vi "IMURead.vi"(10 "baud rate (57600)":u32=57600) -> (3 "Read":string)   [LabVIEW 2017]
uses:
  <vilib>/Instr/_visa.llb/VISA Configure Serial Port (Instr).vi
  <vilib>/Utility/error.llb/Error Cluster From Error Code.vi
  <vilib>/rvi/errors/niLvFpgaAdjustHostInterfaceError.vi
  <vilib>/FPGAPlugInAG/Dynamic/niLvFpga_Close_Dynamic.vi
  <vilib>/rvi/interface/nirviReadWriteControl/nirviReadWriteControl.xnode
  <vilib>/rvi/interface/nirviCloseFPGA/nirviCloseFPGA.xnode
  NiFpgaLv.dll
  <vilib>/rvi/interface/Simulation/niFpgaSimulationCallBeginRW.vi
panel:
  out "Other GSV":sgl
  out "Max Z Accel":sgl
  out "Max Y Accel":sgl
  out "Velocity GSV":dbl
  out "Y Velocity RAW":sgl
  out "Y Accel in m/s^2":sgl
  out "Z dTheta":sgl
  out "Y dTheta":sgl
  out "X dTheta":sgl
  out "Z Accel":sgl
  out "Y Accel":sgl
  out "X Accel":sgl
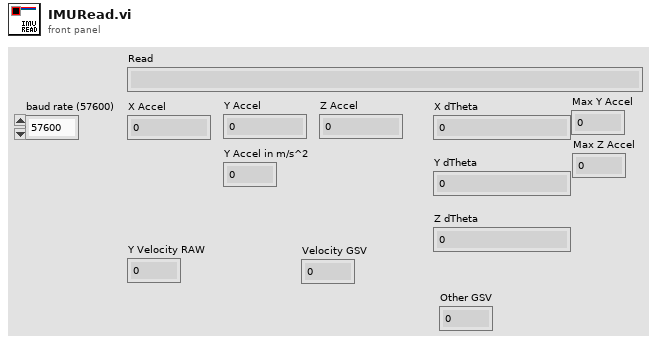
[diagram p1: front panel]
types:
  T1 = cluster{"X dtheta":sgl, "Y dtheta":sgl, "Z dtheta":sgl, "X accel":sgl, "Y accel":sgl, "Z accel":sgl, "Velocity":sgl, "IMU Fault":bool, "Time Since Last Tape":sgl, "Position":sgl}
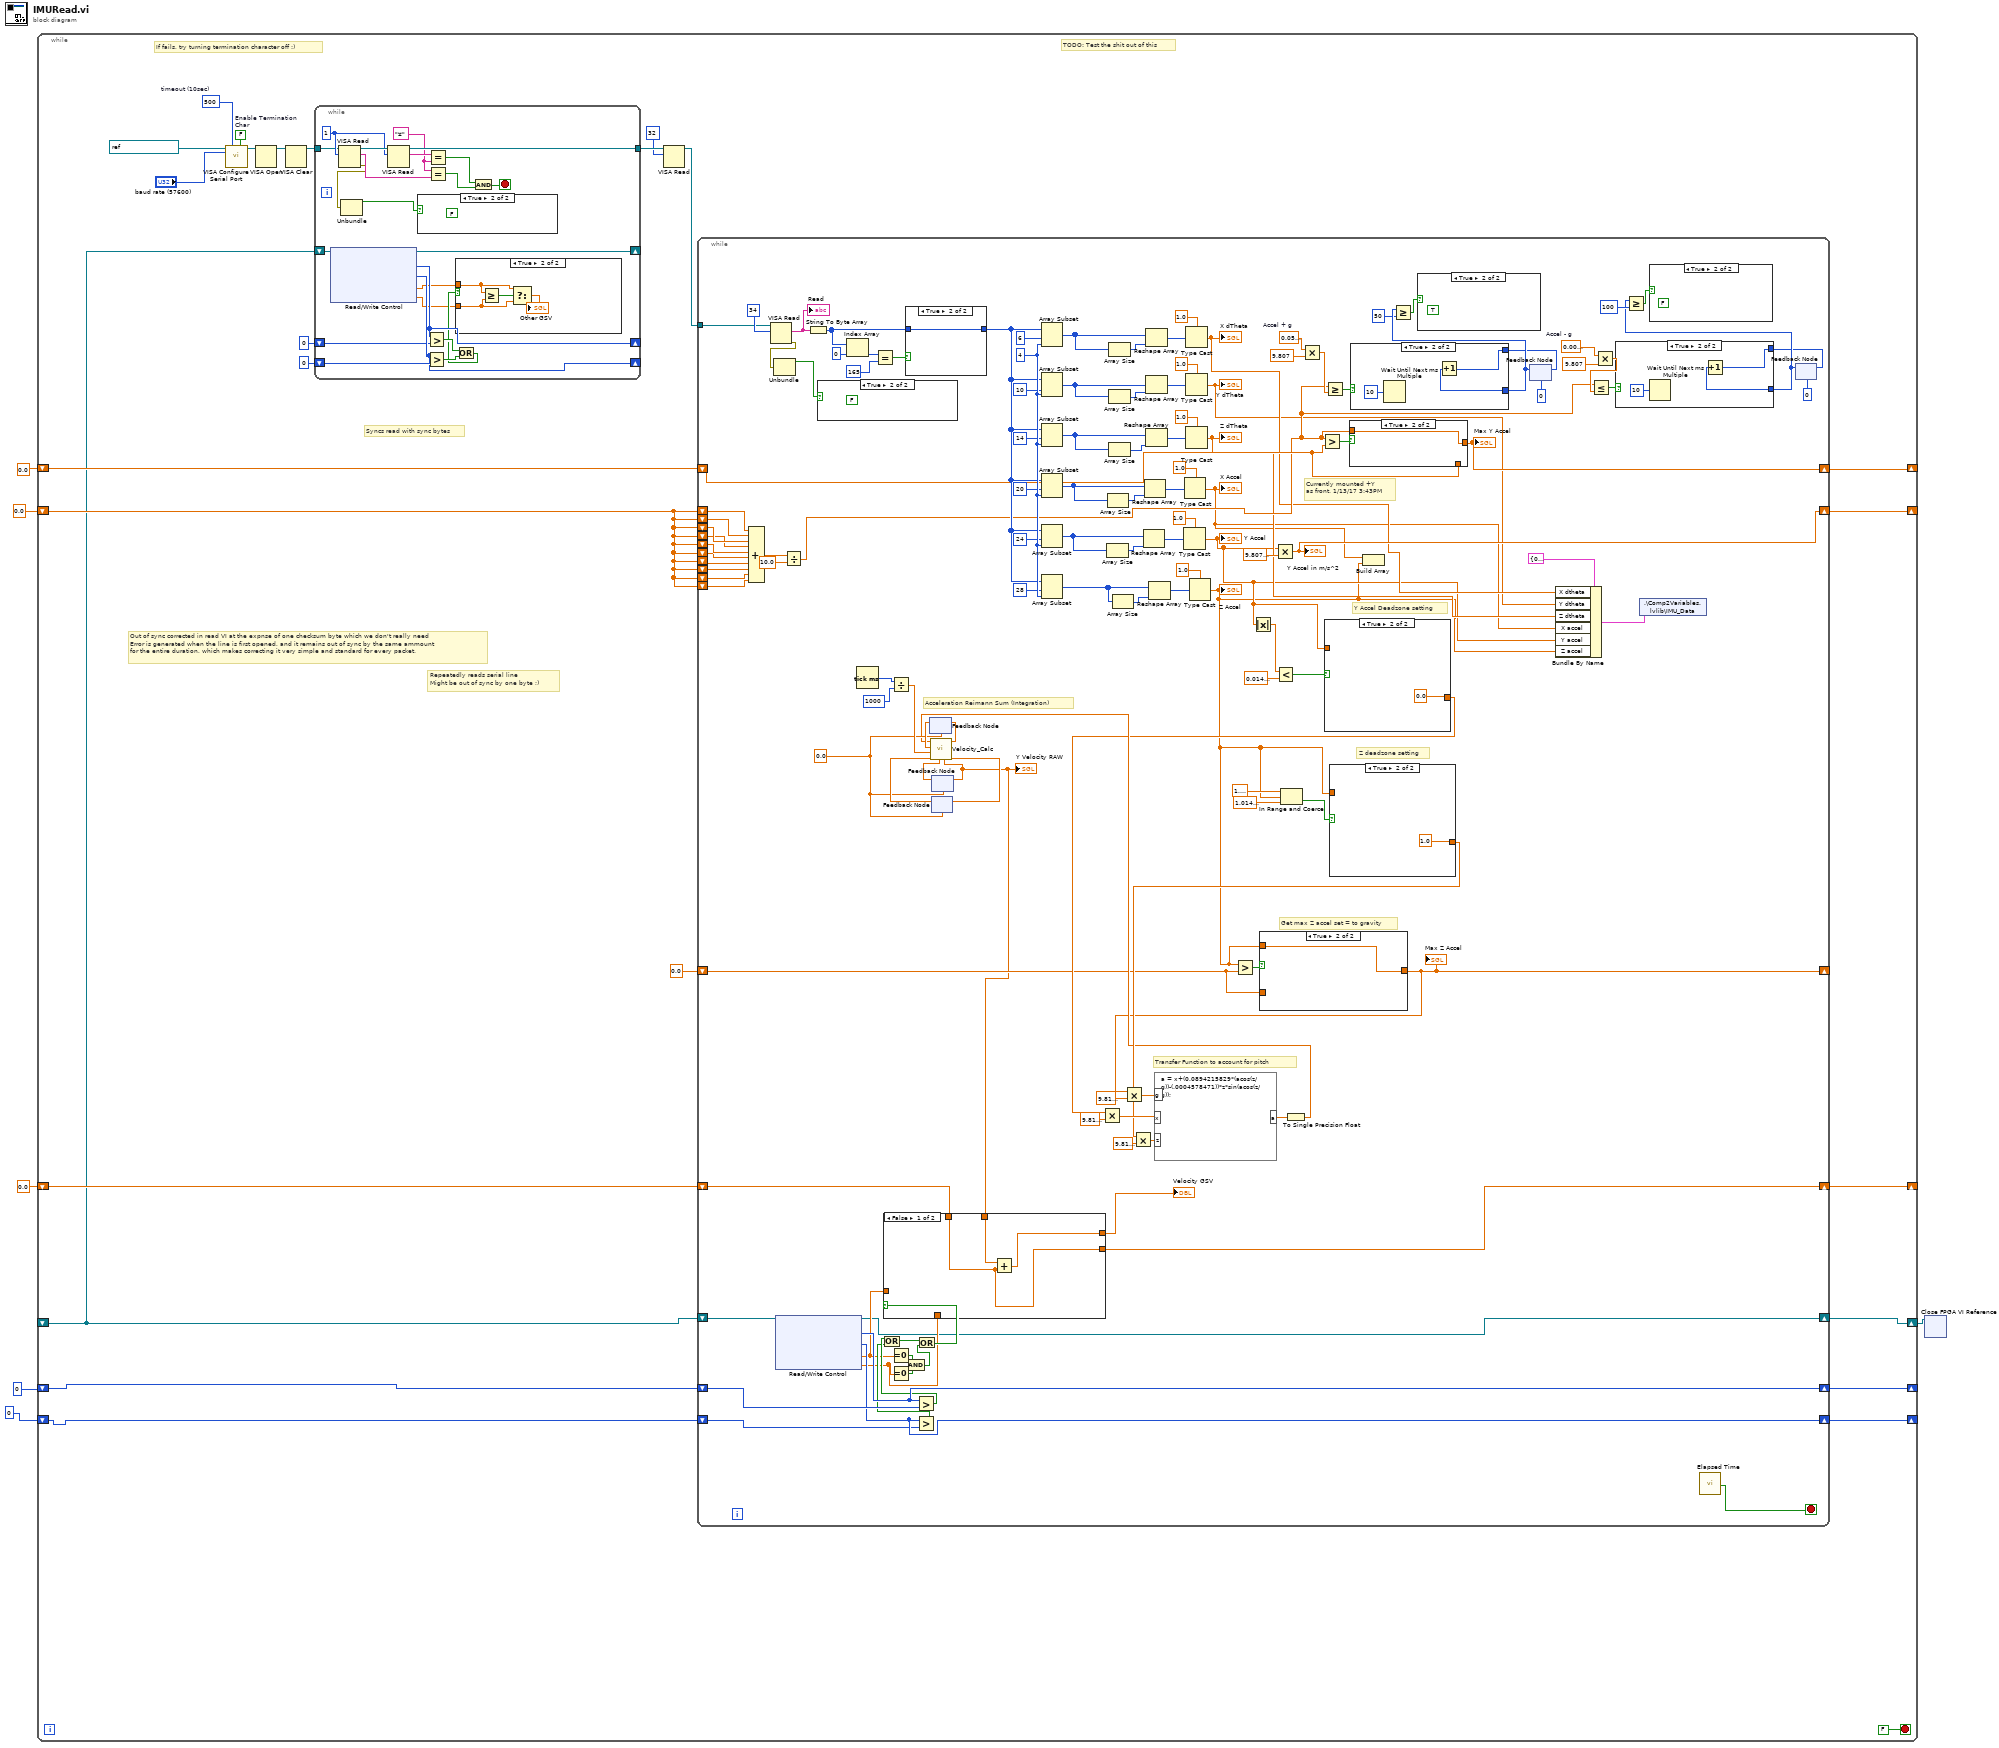
[diagram p0: block diagram]
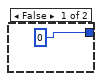
[diagram p4: hidden frame]
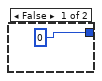
[diagram p6: hidden frame]
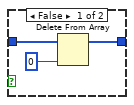
[diagram p9: hidden frame]
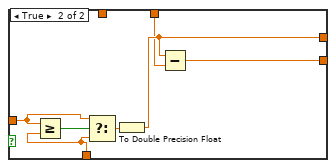
[diagram p10: hidden frame]
diagram:
  n1 = while {
    shift-right: [w23] -> w6
    shift-left: _ -> [w11]
    shift-right: [w22] -> _
    shift-left: u8 0 ("BL Count") -> [w20]
    shift-right: [w21] -> _
    shift-left: u8 0 ("BR Count") -> [w19]
    shift-right: [w17] -> _
    shift-left: sgl 0.0 ("Velocity out") -> [w18]
    shift-right: [w16] -> _
    shift-left: sgl 0.0 -> [w15]
    shift-right: [w12] -> _
    shift-left: sgl 0.0 -> [w13]
    stop <- FALSE stop-if-true
    w7 = u32 500  # timeout (10sec)
    w27 = FALSE  # Enable Termination Char
    # "TODO: Test the shit out of this"
    # "Repeatedly reads serial line\nMight be out of sync by one byte ;)"
    # "Syncs read with sync bytes"
    # "Out of sync corrected in read VI at the expnse of one checksum byte which we don't really need\nError is generated when the line is first opened, and it remains out of sync by the same ammount \nfor the entire duration, which makes correcting it very simple and standard for every packet."
    # "If fails, try turning termination character off :)"
    n2 = call-poly "VISA Configure Serial Port"("VISA resource name"=refnum<visa-resource-name> "ASRL2::INSTR" ("VISA Refnum in"), "timeout (10sec)"=w7, "Enable Termination\nChar (T)"=w27, "baud rate (9600)"="baud rate (57600)") -> ("VISA resource name out"=w8:refnum<visa-resource-name>)  [unwired: 10 in, 1 out]
    n3 = VISA Open(VISA resource name=w8) -> (VISA resource name=w26:refnum<visa-resource-name>)  [unwired: 4 in, 1 out]
    n4 = VISA Clear(VISA resource name=w26) -> (VISA resource name out=w31:refnum<visa-resource-name>)  [unwired: 1 in, 1 out]
    n5 = while {
      tunnel: w31 -> [w199]
      tunnel: [w214] -> w32
      shift-right: [w209] -> _
      shift-left: w11 -> [w210]
      shift-right: [w207] -> _
      shift-left: u8 0 ("BR Count") -> [w208]
      shift-right: [w205] -> _
      shift-left: u8 0 ("BL Count") -> [w206]
      stop <- w211 stop-if-true
      w212 = "¥" ("y")
      w217 = u32 1 ("byte count")
      n6 = xnode "Read/Write Control"("FPGA VI Reference In"=w210) -> ("FPGA VI Reference Out"=w209:refnum<k20>, "BL Count"=w205:u8, "BR Count"=w207:u8, "Velocity Left (m/s)"=w201:sgl, "Velocity Right (m/s)"=w200:sgl)  [unwired: 1 in, 1 out]
      n7 = VISA Read(VISA resource name=w199, byte count=w217) -> (VISA resource name out=w219:refnum<visa-resource-name>, read buffer=w213:string, error out=w198:errorcluster)  [unwired: 1 in, 1 out]
      n8 = Unbundle(w198) -> ("status"=w197:bool)  [unwired: 2 out]
      n9 = VISA Read(VISA resource name=w219, byte count=w217) -> (VISA resource name out=w214:refnum<visa-resource-name>, read buffer=w218:string)  [unwired: 1 in, 2 out]
      n10 = case shown="True" w197 {
        frame False {
        }
        frame True {
          (unwired) FALSE ("IMU Status")
        }
      }
      n11 = Greater?(x=w205, y=w206) -> (0:w204:bool)
      n12 = Greater?(x=w207, y=w208) -> (0:w203:bool)
      n13 = Equal?(x=w218, y=w212) -> (x = y?=w216:bool)
      n14 = Equal?(x=w212, y=w213) -> (x = y?=w215:bool)
      n15 = Or(x=w204, y=w203) -> (x .or. y?=w202:bool)
      n16 = case shown="True" w202 {
        tunnel: w201 -> [_ w222]
        tunnel: w200 -> [_ w221]
        frame False {
        }
        frame True {
          n17 = Greater Or Equal?(x=w222, y=w221) -> (x >= y?=w223:bool)
          n18 = Select(t=w222, s=w223, f=w221) -> (s? t:f=→"Other GSV":sgl)
        }
      }
      n19 = And(x=w216, y=w215) -> (x .and. y?=w211:bool)
    }
    n20 = VISA Read(VISA resource name=w32, byte count=u32 32) -> (VISA resource name out=w30:refnum<visa-resource-name>)  [unwired: 1 in, 3 out]
    n21 = while {
      tunnel: w30 -> [w43]
      shift-right: [w105] -> w17
      shift-left: w18 -> [w106]
      shift-right: [w88] -> w23
      shift-left: w11 -> [w99]
      shift-right: [w98] -> w22
      shift-left: w20 -> [w97]
      shift-right: [w95] -> w21
      shift-left: w19 -> [w94]
      shift-right: [w85] -> w16
      shift-left: w15 -> [w86]
      shift-right: [w80] -> _
      shift-left: sgl 0.0 ("lower limit") -> [w83]
      shift-right: [w45] -> w12
      shift-left: w13 -> [w58]
      shift-left: w13 -> [w57]
      shift-left: w13 -> [w56]
      shift-left: w13 -> [w55]
      shift-left: w13 -> [w54]
      shift-left: w13 -> [w53]
      shift-left: w13 -> [w52]
      shift-left: w13 -> [w51]
      shift-left: w13 -> [w50]
      shift-left: w13 -> [w49]
      stop <- w59 stop-if-true
      w63 = sgl 0.01  # Accel - g
      w67 = sgl 0.05  # Accel + g
      w108 = sgl 0.0 ("Last acceleration out")
      w141 = 4 ("length")
      # "Get max Z accel set = to gravity"
      # "Transfer Function to account for pitch"
      # "Acceleration Reimann Sum (Integration)"
      # "Currently mounted +Y\nas front. 1/13/17 3:43PM"
      # "Z deadzone setting"
      # "Y Accel Deadzone setting"
      n22 = Compound Arithmetic op=ADD(w58, w57, w56, w55, w54, w53, w52, w51, w50, w49) -> (w48:sgl)
      n23 = VISA Read(VISA resource name=w43, byte count=u32 34) -> (read buffer=w60:string, error out=w42:errorcluster)  [unwired: 1 in, 2 out]
      "Read" <- w60
      n24 = Unbundle(w42) -> ("status"=w41:bool)  [unwired: 2 out]
      n25 = xnode "Read/Write Control"("FPGA VI Reference In"=w99) -> ("FPGA VI Reference Out"=w88:refnum<k20>, "BL Count"=w98:u8, "BR Count"=w95:u8, "Velocity Left (m/s)"=w91:sgl, "Velocity Right (m/s)"=w90:sgl)  [unwired: 1 in, 1 out]
      n26 = Divide(x=w48, y=sgl 10.0) -> (x/y=w46:sgl)
      n27 = String To Byte Array(string=w60) -> (unsigned byte array=w137:u8[])
      n28 = case shown="True" w41 {
        frame False {
        }
        frame True {
          (unwired) FALSE ("IMU Status")
        }
      }
      n29 = Index Array(array=w137, index=0) -> (element=w140:u8)
      n30 = Tick Count (ms)() -> (millisecond timer value=w116:u32)
      n31 = Equal?(x=w140, y=u8 165) -> (x = y?=w61:bool)
      n32 = Equal To 0?(x=w91) -> (x = 0?=w104:bool)
      n33 = Equal To 0?(x=w90) -> (x = 0?=w103:bool)
      n34 = Divide(x=w116, y=u32 1000) -> (x/y=w118:sgl)
      n35 = case shown="True" w61 {
        tunnel: w137 -> [w180 w182]
        tunnel: [w179 w182] -> w135
        frame False {
          n36 = Delete From Array(array=w180, index=0) -> (array with subset deleted=w179:u8[])  [unwired: 1 in, 1 out]
        }
        frame True {
        }
      }
      n37 = And(x=w104, y=w103) -> (x .and. y?=w101:bool)
      n38 = Greater?(x=w98, y=w97) -> (0:w96:bool)
      n39 = Greater?(x=w95, y=w94) -> (0:w93:bool)
      n40 = Or(x=w96, y=w93) -> (x .or. y?=w102:bool)
      n41 = Or(x=w102, y=w101) -> (x .or. y?=w100:bool)
      n42 = feedback #1(w108) -> (w124:dbl)
      n43 = feedback #2(w108) -> (w126:dbl)
      n44 = feedback #3(w108) -> (w125:dbl)
      n45 = Array Subset(array=w135, index=6, length=w141) -> (w161:u8[])
      n46 = Array Subset(array=w135, index=10 ("length"), length=w141) -> (w158:u8[])
      n47 = Array Subset(array=w135, index=14, length=w141) -> (w156:u8[])
      n48 = Array Subset(array=w135, index=20, length=w141) -> (w154:u8[])
      n49 = Array Subset(array=w135, index=24, length=w141) -> (w165:u8[])
      n50 = Array Subset(array=w135, index=28, length=w141) -> (w164:u8[])
      n51 = Array Size(array=w165) -> (size(s)=w162:i32)
      n52 = Array Size(array=w154) -> (size(s)=w155:i32)
      n53 = Array Size(array=w161) -> (size(s)=w160:i32)
      n54 = Array Size(array=w158) -> (size(s)=w159:i32)
      n55 = Array Size(array=w156) -> (size(s)=w157:i32)
      n56 = Array Size(array=w164) -> (size(s)=w163:i32)
      n57 = Reshape Array(w165, w162) -> (w150:u8[])
      n58 = Reshape Array(w154, w155) -> (w148:u8[])
      n59 = Reshape Array(w161, w160) -> (w142:u8[])
      n60 = Reshape Array(w158, w159) -> (w144:u8[])
      n61 = Reshape Array(w156, w157) -> (w146:u8[])
      n62 = Reshape Array(w164, w163) -> (w152:u8[])
      n63 = Type Cast(type=sgl 1.0, x=w150) -> (*(type *) &x=w34:sgl)
      "Y Accel" <- w34
      n64 = Type Cast(type=sgl 1.0, x=w148) -> (*(type *) &x=w35:sgl)
      "X Accel" <- w35
      n65 = Type Cast(type=sgl 1.0, x=w142) -> (*(type *) &x=w39:sgl)
      "X dTheta" <- w39
      n66 = Type Cast(type=sgl 1.0, x=w144) -> (*(type *) &x=w38:sgl)
      "Y dTheta" <- w38
      n67 = Type Cast(type=sgl 1.0, x=w146) -> (*(type *) &x=w37:sgl)
      "Z dTheta" <- w37
      n68 = Type Cast(type=sgl 1.0, x=w152) -> (*(type *) &x=w33:sgl)
      "Z Accel" <- w33
      n69 = Greater?(x=w33, y=w83) -> (0:w84:bool)
      n70 = Absolute Value(x=w34) -> (abs(x)=w122:sgl)
      n71 = case shown="True" w84 {
        tunnel: w33 -> [_ w176]
        tunnel: [w175 w176] -> w80
        tunnel: w83 -> [w175 _]
        frame False {
        }
        frame True {
        }
      }
      "Max Z Accel" <- w80
      n72 = Multiply(x=w80, y=sgl 9.81) -> (x*y=w81:sgl)
      n73 = Multiply(x=w34, y=sgl 9.807) -> (x*y=w45:sgl)
      "Y Accel in m/s^2" <- w45
      n74 = Less?(x=w122, y=sgl 0.015) -> (x < y?=w119:bool)
      n75 = In Range and Coerce(upper limit=sgl 1.2, x=w33, lower limit=sgl 1.015) -> (In Range?=w110:bool)  [unwired: 1 out]
      n76 = Multiply(x=w67, y=9.807) -> (x*y=w65:dbl)
      n77 = Greater?(x=w46, y=w86) -> (0:w87:bool)
      n78 = Greater Or Equal?(x=w46, y=w65) -> (x >= y?=w78:bool)
      n79 = case shown="True" w119 {
        tunnel: [w195 sgl 0.0 ("Acceleration")] -> w89
        tunnel: w34 -> [w195 _]
        frame False {
        }
        frame True {
        }
      }
      n80 = Multiply(x=w89, y=sgl 9.81) -> (x*y=w112:sgl)
      n81 = case shown="True" w110 {
        tunnel: [w193 sgl 1.0 ("Acceleration")] -> w109
        tunnel: w33 -> [w193 _]
        frame False {
        }
        frame True {
        }
      }
      n82 = Multiply(x=w109, y=sgl 9.81) -> (x*y=w114:sgl)
      n83 = formula code="a = x+(0.0894215829*(acos(z/g))-(.0004578471))*z*sin(acos(z/g));"("x"=w112, "z"=w114, "g"=w81) -> ("a"=w111:dbl)
      n84 = To Single Precision Float(number=w111) -> (single precision float=w107:sgl)
      n85 = call "Velocity_Calc.vi"("Velocity in"=w125, "Last time in"=w126, "Time"=w118, "Last acceleration in"=w124, "Acceleration"=w107) -> ("Last time out"=w127:dbl, "Last acceleration out"=w128:dbl, "Velocity out"=w44:dbl)  [unwired: 4 in]
      "Y Velocity RAW" <- w44
      n86 = case shown="False" w100 {
        tunnel: [w185 w187] -> w92
        tunnel: w106 -> [w184 _]
        tunnel: [w184 w192] -> w105
        tunnel: w91 -> [_ w189]
        tunnel: w90 -> [_ w188]
        tunnel: w44 -> [w183 w186]
        frame False {
          n87 = Add(x=w183, y=w184) -> (x+y=w185:dbl)
        }
        frame True {
          n88 = Greater Or Equal?(x=w189, y=w188) -> (x >= y?=w191:bool)
          n89 = Select(t=w189, s=w191, f=w188) -> (s? t:f=w190:sgl)
          n90 = To Double Precision Float(number=w190) -> (double precision float=w187:dbl)
          n91 = Subtract(x=w187, y=w186) -> (x-y=w192:dbl)
        }
      }
      "Velocity GSV" <- w92
      n92 = feedback-in #1(w128) -> ()
      n93 = feedback-in #2(w127) -> ()
      n94 = feedback-in #3(w44) -> ()
      n95 = case shown="True" w87 {
        tunnel: [w177 w178] -> w85
        tunnel: w86 -> [w177 _]
        tunnel: w46 -> [_ w178]
        frame False {
        }
        frame True {
        }
      }
      "Max Y Accel" <- w85
      n96 = Build Array(w35, w33) -> ()  [unwired: 1 out]
      n97 = feedback #4(u32 0 ("milliseconds to wait")) -> (w77:u32)
      n98 = case shown="True" w78 {
        tunnel: [u32 0 ("milliseconds to wait") w173] -> w75
        tunnel: w77 -> [_ w172]
        frame False {
        }
        frame True {
          n99 = Wait Until Next ms Multiple(millisecond multiple=u32 10 ("milliseconds to wait")) -> ()  [unwired: 1 out]
          n100 = Increment(x=w172) -> (x+1=w173:u32)
        }
      }
      n101 = Greater Or Equal?(x=w77, y=u32 50) -> (x >= y?=w74:bool)
      n102 = case shown="True" w74 {
        frame False {
        }
        frame True {
          (unwired) TRUE
        }
      }
      n103 = feedback-in #4(w75) -> ()
      n104 = Bundle By Name(cluster=T1 {"X dtheta"=0.0, "Y dtheta"=0.0, "Z dtheta"=0.0, "X accel"=0.0, "Y accel"=0.0, "Z accel"=0.0, "Velocity"=0.0, "IMU Fault"=FALSE, "Time Since Last Tape"=0.0, "Position"=0.0} ("IMU_Data"), "X dtheta"=w39, "Y dtheta"=w38, "Z dtheta"=w37, "X accel"=w35, "Y accel"=w34, "Z accel"=w33) -> (w36:T1)
      n105 = Multiply(x=w63, y=9.807) -> (x*y=w62:dbl)
      n106 = Less Or Equal?(x=w46, y=w62) -> (x <= y?=w73:bool)
      n107 = shared-variable ".\\Comp2Variables.lvlib\\IMU_Data"(w36) -> ()  [unwired: 1 in, 1 out]
      n108 = call "Elapsed Time"() -> ("Time has Elapsed"=w59:bool)  [unwired: 12 in, 7 out]
      n109 = feedback #5(u32 0 ("milliseconds to wait")) -> (w69:u32)
      n110 = case shown="True" w73 {
        tunnel: [u32 0 ("milliseconds to wait") w169] -> w68
        tunnel: w69 -> [_ w168]
        frame False {
        }
        frame True {
          n111 = Wait Until Next ms Multiple(millisecond multiple=u32 10 ("milliseconds to wait")) -> ()  [unwired: 1 out]
          n112 = Increment(x=w168) -> (x+1=w169:u32)
        }
      }
      n113 = Greater Or Equal?(x=w69, y=u32 100) -> (x >= y?=w71:bool)
      n114 = case shown="True" w71 {
        frame False {
        }
        frame True {
          (unwired) FALSE
        }
      }
      n115 = feedback-in #5(w68) -> ()
    }
  }
  n116 = xnode "Close FPGA VI Reference"("FPGA VI Reference In"=w6) -> ()  [unwired: 1 in, 1 out]
